vi "Set Input Muted.vi"(8 "error in (no error)":errorcluster, 9 "Muted":bool, 10 "Input Name":string, 11 "OBS in":refnum<class "OBS.lvclass">) -> (0 "error out":errorcluster, 3 "OBS out":refnum<class "OBS.lvclass">)   [LabVIEW 2020, in "obs-websocket.lvlib" / "OBS.lvclass"]
uses:
  OBS.lvclass
  OBS.lvclass/OBS.ctl
  SetInputMute/SetInputMute.lvclass
  C:/dev/lv20CE/lv-obs-websocket/obs-websocket-lv/Request/Request.lvclass
  C:/dev/lv20CE/lv-obs-websocket/obs-websocket-lv/Client Message/Client Message.lvclass
  C:/dev/lv20CE/lv-obs-websocket/obs-websocket-lv/Message/Message.lvclass
  C:/dev/lv20CE/lv-obs-websocket/obs-websocket-lv/SetInputMute/SetInputMute.lvclass
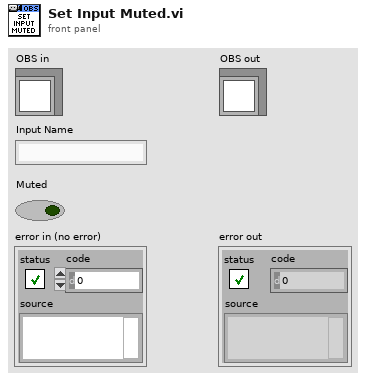
[diagram p1: front panel]
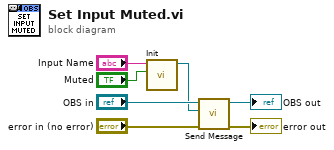
[diagram p0: block diagram]
diagram:
  n1 = call "Init.vi"("Muted"="Muted", "Input Name"="Input Name") -> ("SetInputMute out"=w5:refnum<class "SetInputMute.lvclass">)  [unwired: 8 in, 1 out]
  n2 = call "Send Message.vi"("error in (no error)"="error in (no error)", "Client Message"=w5, "OBS in"="OBS in") -> ("error out"=→"error out":errorcluster, "OBS in"=→"OBS out":refnum<class "OBS.lvclass">)  [unwired: 5 in, 2 out]
